vi "Initialize Attributes.vi"(8 "error in (no error)":errorcluster, 10 "Attribute Data":variant, 11 "CS++DSCAlarmViewer in":refnum<class "CS++DSCAlarmViewer.lvclass">) -> (0 "error out":errorcluster, 2 "Found?":bool, 3 "CS++DSCAlarmViewer out":refnum<class "CS++DSCAlarmViewer.lvclass">)   [LabVIEW 2016, in "CS++DSCAlarmViewer.lvlib" / "CS++DSCAlarmViewer.lvclass"]
doc: "Initialize object attribute.\n\nUnique resources should be allocated elsewhere!"
uses:
  CS++DSCAlarmViewer.lvclass
  CS++DSCAlarmViewer.lvclass/CS++DSCAlarmViewer.ctl
  CSPP_Core/Actors/CS++GUIActor/CS++GUIActor.lvclass
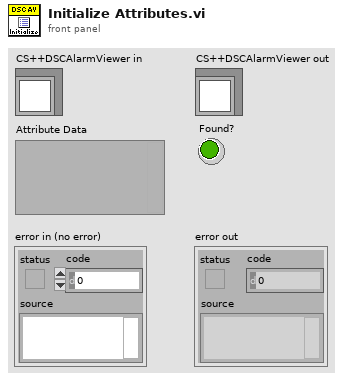
[diagram p1: front panel]
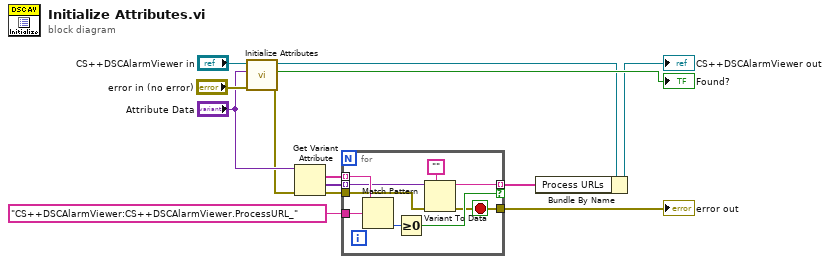
[diagram p0: block diagram]
diagram:
  n1 = call-parent "Initialize Attributes.vi"("error in (no error)"="error in (no error)", "Attribute Data"="Attribute Data", "CS++GUIActor in"="CS++DSCAlarmViewer in") -> ("error out"=w9:errorcluster, "Found?"=→"Found?":bool, "CS++GUIActor out"=w3:refnum<class "CS++DSCAlarmViewer.lvclass">)  [unwired: 6 in]
  n2 = Get Variant Attribute(Variant="Attribute Data", error in=w9) -> (names=w8:string[], values=w7:variant[], error out=w6:errorcluster)  [unwired: 2 in, 1 out]
  n3 = for {
    tunnel: w8 -> [w22] mode=indexing
    tunnel: w7 -> [w19] mode=indexing
    tunnel: w6 -> [w17]
    tunnel: "CS++DSCAlarmViewer:CS++DSCAlarmViewer.ProcessURL_" -> [w21]
    tunnel: [w16] -> w1 mode=indexing if=w15
    tunnel: [w14] -> w4
    stop <- w14 stop-if-true
    n4 = Match Pattern(string=w22, regular expression=w21) -> (offset past match=w20:i32)  [unwired: 1 in, 3 out]
    n5 = Greater Or Equal To 0?(x=w20) -> (x >= 0?=w15:bool)
    n6 = Variant To Data(error in=w17, type="", Variant=w19) -> (data=w16:string, error out=w14:errorcluster)
  }
  "error out" <- w4
  n7 = Bundle By Name(cluster=w3, "Process URLs"=w1) -> (→"CS++DSCAlarmViewer out":refnum<class "CS++DSCAlarmViewer.lvclass">)
